vi "HackRF_SetGain_Rx.vi"(7 "AMPEnable":bool, 8 "error in (no error)":errorcluster, 9 "VGAGainDb":dbl min=0.0 max=62.0 step=2.0, 10 "LNAGainDb":dbl min=0.0 max=40.0 step=8.0, 11 "HackRF in":T1) -> (0 "error out":errorcluster, 3 "HackRF out":T1)   [LabVIEW 2021]
doc: "The three RX gain controls are at the RF (\"amp\", 0 or 14 dB), IF gain (\"lna\", 0 to 40 dB in 8 dB steps), and baseband (\"vga\", 0 to 62 dB in 2 dB steps) stages."
uses:
  HackRF_Ref.ctl
  C:/Program Files/HackRF/labview/NetHackrf.dll
  NetHackrf.dll
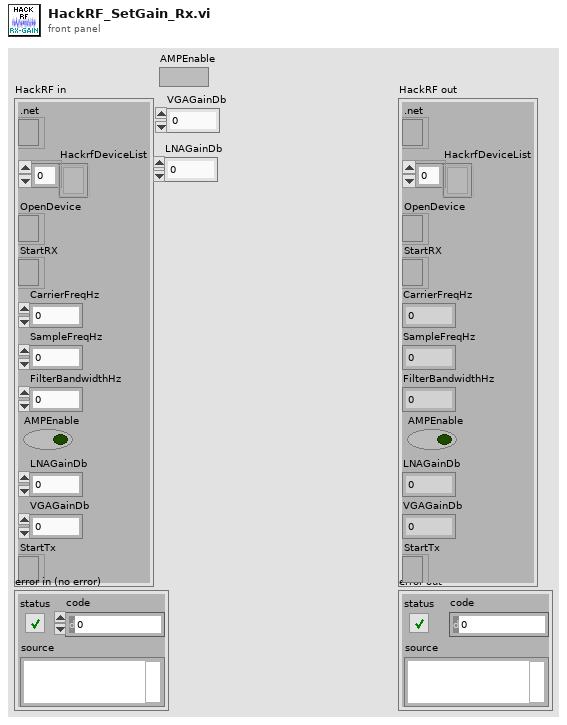
[diagram p1: front panel]
types:
  T1 = typedef "HackRF_Ref.ctl" = cluster{".net":refnum<k24>, "HackrfDeviceList":refnum<k24>[], "OpenDevice":refnum<k24>, "StartRX":refnum<k24>, "CarrierFreqHz":dbl, "SampleFreqHz":dbl, "FilterBandwidthHz":dbl, "AMPEnable":bool, "LNAGainDb":dbl, "VGAGainDb":dbl, "StartTx":refnum<k24>}
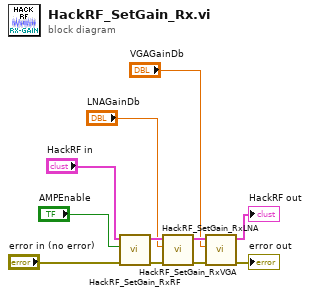
[diagram p0: block diagram]
diagram:
  n1 = call "HackRF_SetGain_RxRF.vi"("error in (no error)"="error in (no error)", "AMPEnable"="AMPEnable", "HackRF in"="HackRF in") -> ("error out"=w11:errorcluster, "HackRF out"=w10:T1)  [unwired: 7 in]
  n2 = call "HackRF_SetGain_RxLNA.vi"("error in (no error)"=w11, "LNAGainDb"="LNAGainDb", "HackRF in"=w10) -> ("error out"=w9:errorcluster, "HackRF out"=w8:T1)  [unwired: 7 in]
  n3 = call "HackRF_SetGain_RxVGA.vi"("error in (no error)"=w9, "VGAGainDb"="VGAGainDb", "HackRF in"=w8) -> ("error out"=→"error out":errorcluster, "HackRF out"=→"HackRF out":T1)  [unwired: 7 in]
